vi "Create Instructions Channel.vi"(8 "error in (no error)":errorcluster) -> (0 "error out":errorcluster, 3 "Instructions":refnum<user-event>)   [LabVIEW 2020, in "RTAF.lvlib" / "Actor.lvclass"]
uses:
  Actor.lvclass
  Message.ctl
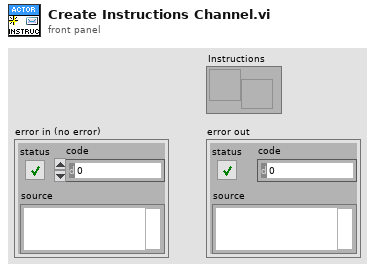
[diagram p1: front panel]
types:
  T1 = typedef "RTAF.lvlib/Actor.lvclass/Message.ctl" = cluster{"Name":string, "Payload":variant, "Response Channel":refnum<notifier>}
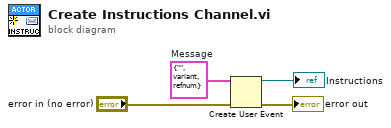
[diagram p0: block diagram]
diagram:
  w4 = T1 {"Name"="", "Payload"=variant, "Response Channel"=refnum}  # Message
  n1 = Create User Event(user event datatype=w4, error in="error in (no error)") -> (user event=→"Instructions":refnum<user-event>, error out=→"error out":errorcluster)
